vi "AB_API Get Destinations.vi"(8 "error in (no error)":errorcluster, 11 "Build in":refnum<class "AB_Build.lvclass">) -> (0 "error out":errorcluster, 2 "Destinations":T1[](array[typedef]))   [LabVIEW 2020]
uses:
  <vilib>/AppBuilder/AB_Classes/Build/AB_Build.lvclass
  <vilib>/AppBuilder/AB_API/common/AB_API Destination Data.ctl
  <vilib>/AppBuilder/AB_API/common/AB_API Destination Type.ctl
  <vilib>/AppBuilder/AB_Classes/Destination/AB_Destination.lvclass
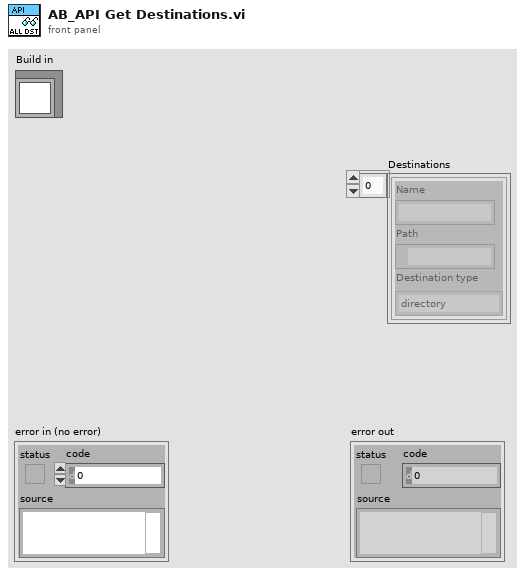
[diagram p1: front panel]
types:
  T1 = typedef "AB_API Destination Data.ctl" = cluster{"Name":string, "Path":path, "Destination type":T2}
  T2 = typedef "AB_API Destination Type.ctl" = enum16{"directory", "directory (preserve hierarchy)", "LLB"}
  T3 = typedef "AB_Build.ctl" = cluster{"buildSpecName":string, "buildSpecDescription":string, "destinations":refnum<class "AB_Destination.lvclass">[], "exclusionOption":T4, "defaultLanguage":string, "supportedLanguages":string[], "excludedDirectories":path[], "buildContext":refnum<vi>, "buildObject":T5, "preview":bool, "programatic":bool, "progressBarEvents":T6, "userLog_Path":path, "preActionID":string, "preAction_Path":path, "postActionID":string, "postAction_Path":path, "eng_checkForBrokenVIs?":bool, "eng_verboseLinkerErrors?":bool, "localDest_Path":path, "targetDest_Path":path, "removeVIObject":u16, "cache":refnum<class "PreviewCache.lvclass">, "use cache":bool, "previewCache_ID":string, "buildCache_ID":string, "eng_TempLocalDest_Path":path, "eng_collectDependencies?":bool, "versionInfo":cluster{"buildVersion":cluster{"major":u16, "minor":u16, "patch":u16, "build":u16}, "autoIncrement":bool}, "eng_enableVIChecksums":bool}
  T4 = typedef "AB_Exclusion_Option.ctl" = cluster{"typedefs":bool, "polymorphicVIs":bool, "unusedLibraryItems":bool, "modifyLibraryFile":bool, "edit-timeDependencies":bool, "inlineVIs":bool, "dependent PPLs":bool, "dependent DLLs":bool}
  T5 = typedef "ItemRef.ctl" = u64
  T6 = typedef "provcom_ProgressBar_Events.ctl" = cluster{"newJob":refnum<user-event>, "newItem":refnum<user-event>, "errorMsg":T7, "cancel":refnum<user-event>}
  T7 = typedef "mxLvBuildError.ctl" = refnum<user-event>
  T8 = typedef "AB_Destination.ctl" = cluster{"destName":string, "path":path, "libraryName":string, "preserveHierarchy":bool, "eng_inBuild":bool, "eng_libraryReference":refnum<vi>, "eng_restictAddToNewLibrary":bool}
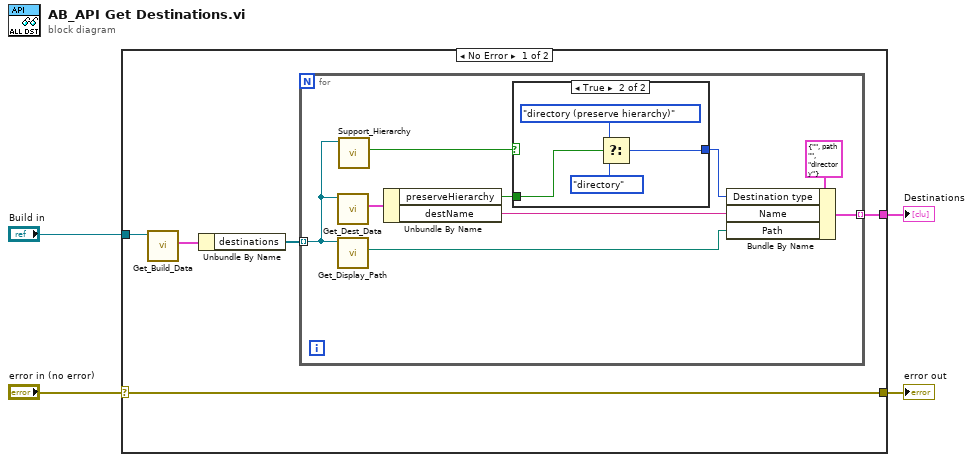
[diagram p0: block diagram]
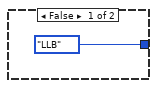
[diagram p2: hidden frame]
diagram:
  n1 = case shown="No Error" "error in (no error)" {
    selector: "error in (no error)" -> [w9 w24]
    tunnel: [w9 w24] -> w3
    tunnel: "Build in" -> [w7 _]
    tunnel: [w5 _] -> w1
    frame No Error {
      n2 = call <vilib>:"Get_Build_Data.vi"("Class in"=w7) -> ("data"=w8:T3)  [unwired: 1 in, 9 out]
      n3 = Unbundle By Name(w8) -> ("destinations"=w6:refnum<class "AB_Destination.lvclass">[])
      n4 = for {
        tunnel: w6 -> [w14] mode=indexing
        tunnel: [w16] -> w5 mode=indexing
        n5 = call <vilib>:"Get_Dest_Data.vi"("Class in"=w14) -> ("destName"=w18:T8)  [unwired: 8 in, 2 out]
        n6 = call-dynamic "Get_Display_Path.vi"("AB_Destination in"=w14) -> ("displayPath"=w15:path)  [unwired: 1 in, 9 out]
        n7 = call-dynamic "Support_Hierarchy.vi"("AB_Destination in"=w14) -> ("support hierarchy"=w13:bool)  [unwired: 8 in, 2 out]
        n8 = Unbundle By Name(w18) -> ("preserveHierarchy"=w11:bool, "destName"=w12:string)
        n9 = case shown="True" w13 {
          tunnel: [AB_API_Destination_Type."LLB" ("Destination type") w21] -> w10
          tunnel: w11 -> [_ w23]
          frame False {
          }
          frame True {
            n10 = Select(t=AB_API_Destination_Type."directory (preserve hierarchy)" ("Destination type"), s=w23, f=AB_API_Destination_Type."directory" ("Destination type")) -> (s? t:f=w21:T2)
          }
        }
        n11 = Bundle By Name(cluster=T1 {"Name"="", "Path"=path "", "Destination type"=enum."directory"} ("Destination Data"), "Destination type"=w10, "Name"=w12, "Path"=w15) -> (w16:T1)
      }
    }
    frame Error {
    }
  }
  "error out" <- w3
  "Destinations" <- w1
